vi "JibeSailSuggestion.vi"(4 "OLD Suggested Rudder Setpoint":T1 min=-1.0 max=1.0, 6 "OLD Suggested Sail Setpoints":T2 {"MainSailSuggestion" min=0.0 max=1.0; "JibSailSuggestion" min=0.0 max=1.0}, 8 "DesiredHeading":dbl, 9 "WindSpeed":dbl, 10 "RobotHeading":dbl, 11 "AbsoluteWindAngle":dbl) -> (2 "Suggested Rudder Setpoint":T1 min=-1.0 max=1.0, 3 "Suggested Sail Setpoints":T2 {"MainSailSuggestion" min=0.0 max=1.0; "JibSailSuggestion" min=0.0 max=1.0})   [LabVIEW 2012]
doc: "This VI should output sail and rudder instructions for how to jibe across the wind. Inputs could include wind direction, robot heading, desired heading, and others of interest. Algorithm currently undetermined, ask sailors for jibe thought process and communicate with the forebrain programmers to figure out when the boat will be considered in a jibe and when it will be considered out of one. See TackingSailSuggestion.vi for comparison."
uses:
  Data/TypeDefs/Sail Set Suggestions.ctl
  Data/TypeDefs/Rudder Set Suggestions.ctl
panel:
  # "This VI should output sail and rudder instructions for how\nto jibe across the wind. Inputs could include wind direction,\nrobot heading, desired heading, and others of interest.\nAlgorithm currently undetermined, ask sailors for jibe\nthought process and communicate with the forebrain\nprogrammers to figure out when the boat will be considered\nin a jibe and when it will be considered out of one. See\nTackingSailSuggestion.vi for comparison."
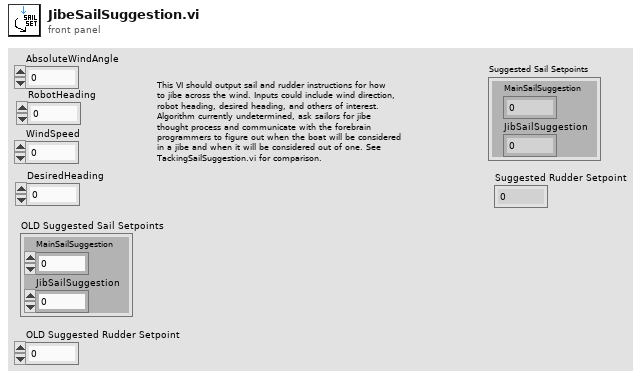
[diagram p1: front panel]
types:
  T1 = typedef "Rudder Set Suggestions.ctl" = dbl
  T2 = typedef "Sail Set Suggestions.ctl" = cluster{"MainSailSuggestion":dbl, "JibSailSuggestion":dbl}
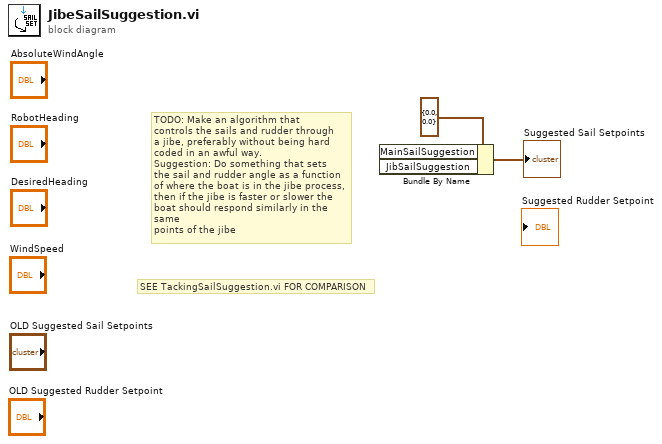
[diagram p0: block diagram]
diagram:
  # "SEE TackingSailSuggestion.vi FOR COMPARISON"
  # "TODO: Make an algorithm that\ncontrols the sails and rudder through\na jibe, preferably without being hard\ncoded in an awful way.\nSuggestion: Do something that sets\nthe sail and rudder angle as a function\nof where the boat is in the jibe process,\nthen if the jibe is faster or slower the\nboat should respond similarly in the same\npoints of the jibe"
  n1 = Bundle By Name(cluster=T2 {"MainSailSuggestion"=0.0, "JibSailSuggestion"=0.0} ("output cluster")) -> (→"Suggested Sail Setpoints":T2)  [unwired: 2 in]
